vi "getScope.vi"(8 "error in (no error)":errorcluster, 11 "tBSONJavaScriptWithScope in":refnum<class "tBSONJavaScriptWithScope.lvclass">) -> (0 "error out":errorcluster, 2 "Scope":refnum<class "tBSONDocument.lvclass">, 3 "tBSONJavaScriptWithScope out":refnum<class "tBSONJavaScriptWithScope.lvclass">)   [LabVIEW 2013, in "BSON.lvlib" / "tBSONJavaScriptWithScope.lvclass"]
uses:
  tBSONJavaScriptWithScope.lvclass
  tBSONDocument/tBSONDocument.lvclass
  tBSONJavaScriptWithScope.lvclass/tBSONJavaScriptWithScope.ctl
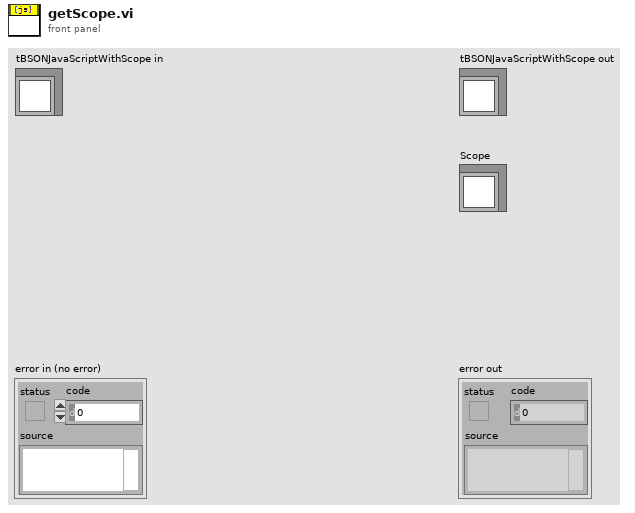
[diagram p1: front panel]
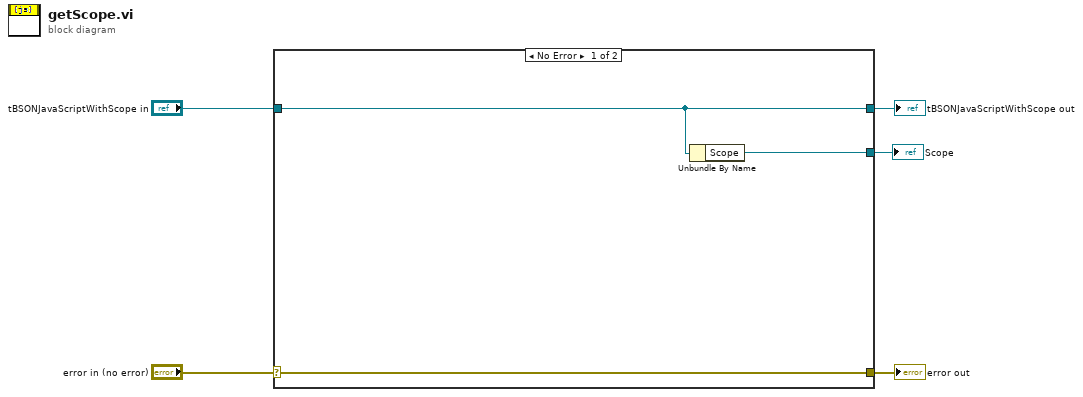
[diagram p0: block diagram]
diagram:
  n1 = case shown="No Error" "error in (no error)" {
    selector: "error in (no error)" -> [w8 w10]
    tunnel: [w8 w10] -> w4
    tunnel: [w7 w9] -> w2
    tunnel: "tBSONJavaScriptWithScope in" -> [w7 w9]
    tunnel: [w6 _] -> w1
    frame No Error {
      n2 = Unbundle By Name(w7) -> ("Scope"=w6:refnum<class "tBSONDocument.lvclass">)
    }
    frame Error {
    }
  }
  "error out" <- w4
  "tBSONJavaScriptWithScope out" <- w2
  "Scope" <- w1
